vi "MB_TCP_ZERO.vi"(5 "Status Reference":T1, 6 "N":i32, 7 "Data Reference":T2, 9 "timeouts":T3={"conn_timeout"=1000, "reconn_timeout"=3000, "N attempt max"=3, "t_reset_TTL"=120000, "write_timeout"=10, "read_timeout"=500, "period"=100} {"t_reset_TTL" min=10 max=240000 step=1; "period" min=10 max=100000 step=1; "read_timeout" min=10 max=60000 step=1; "write_timeout" min=1 max=60000 step=1; "N attempt max" min=1 max=5 step=1; "reconn_timeout" min=10 max=240000 step=1; "conn_timeout" min=10 max=240000}, 10 "write enable":bool=TRUE, 11 "stop":bool) -> (0 "error out":errorcluster, 2 "errors":i32, 3 "Z3":u32)   [LabVIEW 2019, in "MB_TCP1.lvlib"]
uses:
  MB_TCP1.lvlib
  ICPCON Registers/Ctl/ICPCON Data.ctl
  ICPCON Status/Ctl/ICPCON Status.ctl
  Timer Delay/unix time 1ms.vi
  Timer Delay/Timers.lvlib
  ICPCON Registers/ICPCON Registers.lvlib
  ICPCON Status/ICPCON Status.lvlib
panel:
  out "stopped":bool
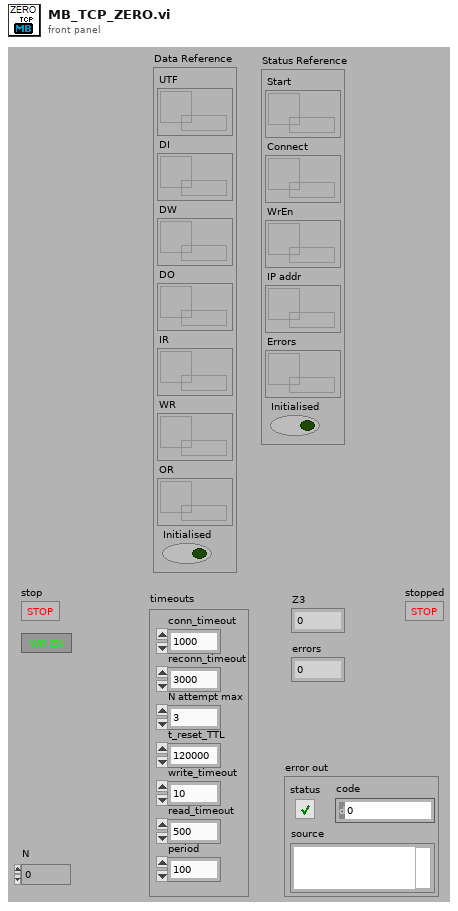
[diagram p1: front panel]
types:
  T1 = typedef "ICPCON Status.lvlib/ICPCON Status.ctl" = cluster{"Start":refnum<data-value>, "Connect":refnum<data-value>, "WrEn":refnum<data-value>, "IP addr":refnum<data-value>, "Errors":refnum<data-value>, "Initialised":bool}
  T2 = typedef "ICPCON Registers.lvlib/ICPCON Data.ctl" = cluster{"UTF":refnum<data-value>, "DI":refnum<data-value>, "DW":refnum<data-value>, "DO":refnum<data-value>, "IR":refnum<data-value>, "WR":refnum<data-value>, "OR":refnum<data-value>, "Initialised":bool}
  T3 = cluster{"conn_timeout":i32, "reconn_timeout":i32, "N attempt max":i32, "t_reset_TTL":i32, "write_timeout":i32, "read_timeout":i32, "period":i32}
  T4 = cluster{"Remote IP Address":string, "Remote Port":u16}
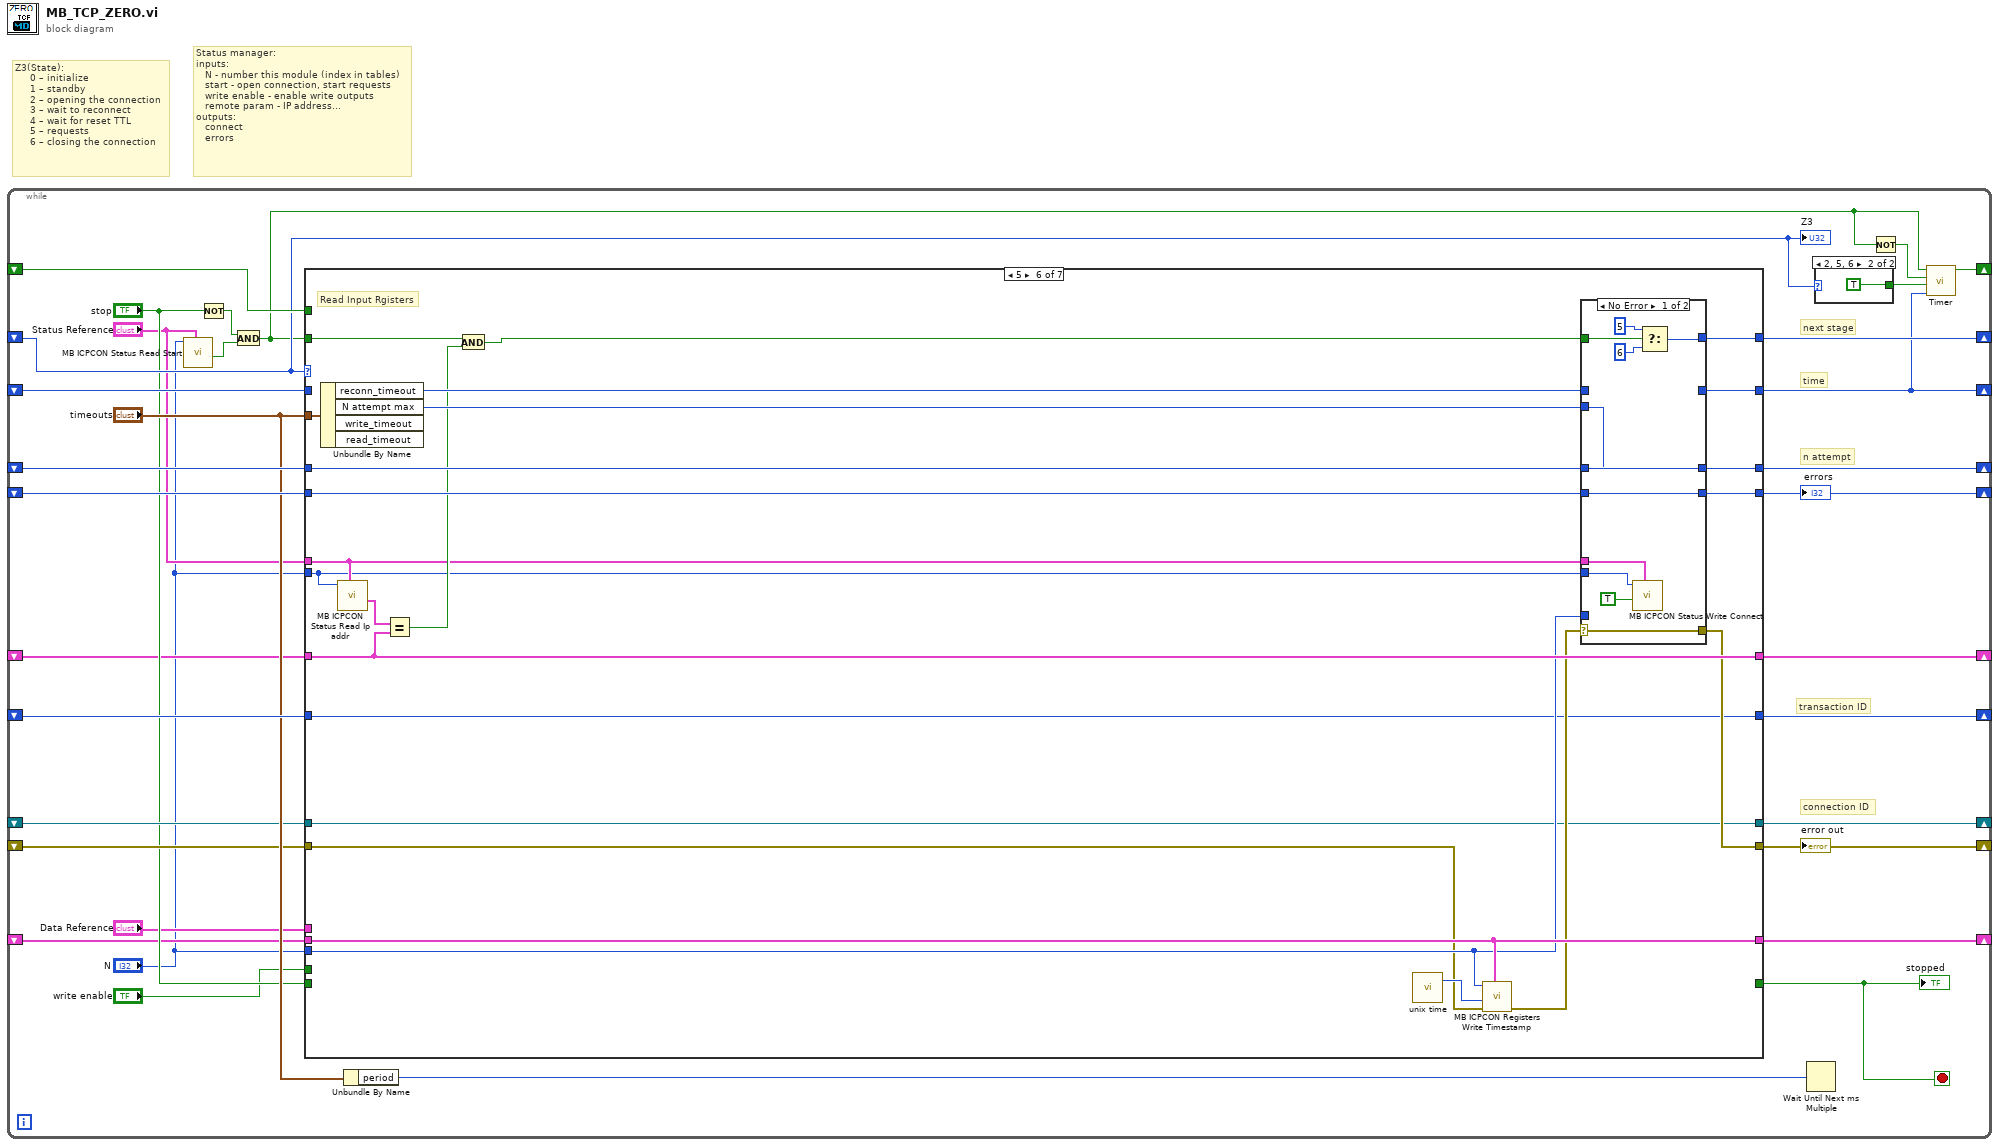
[diagram p0: block diagram]
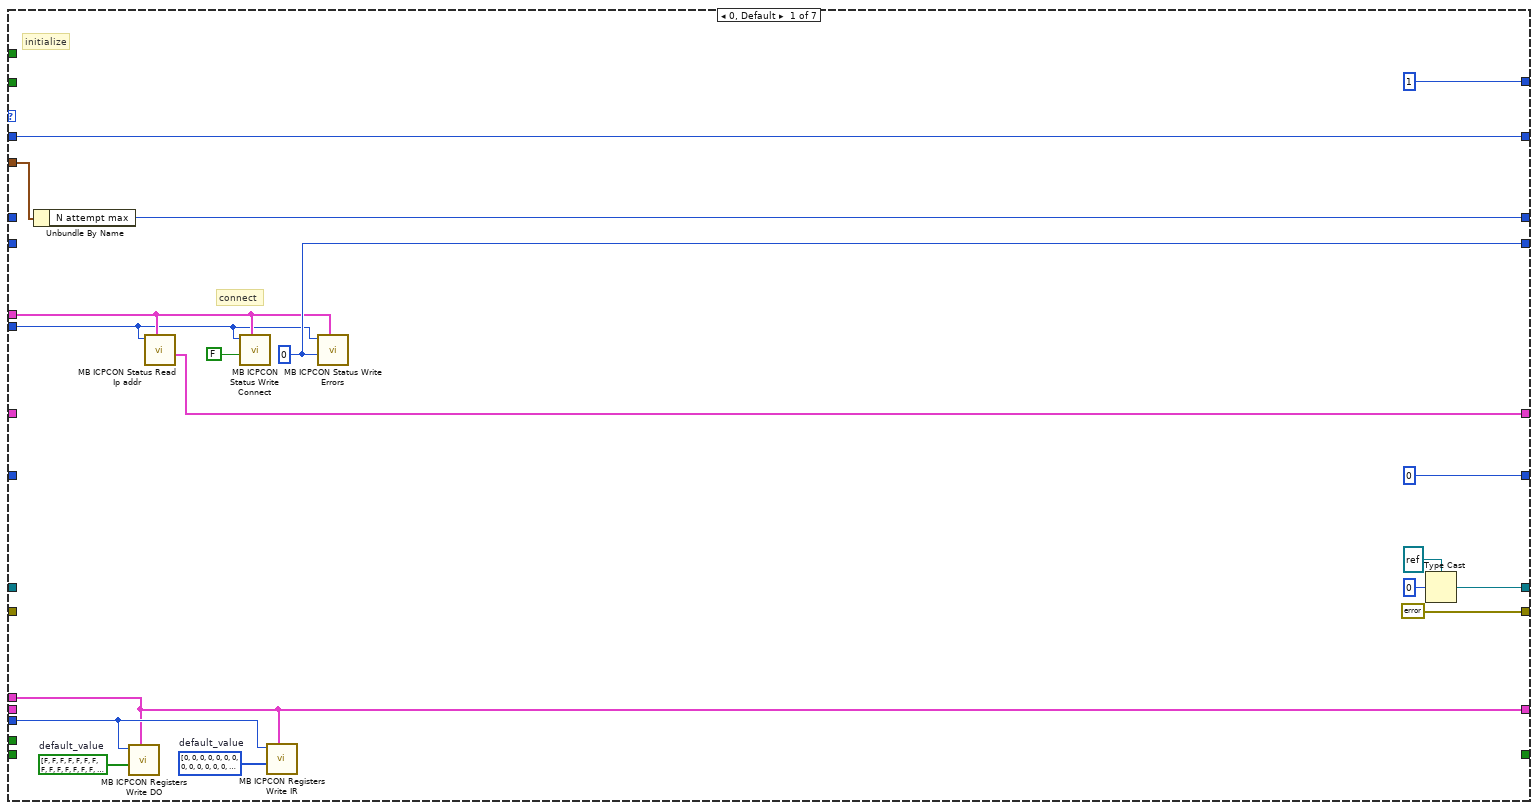
[diagram p2: hidden frame]
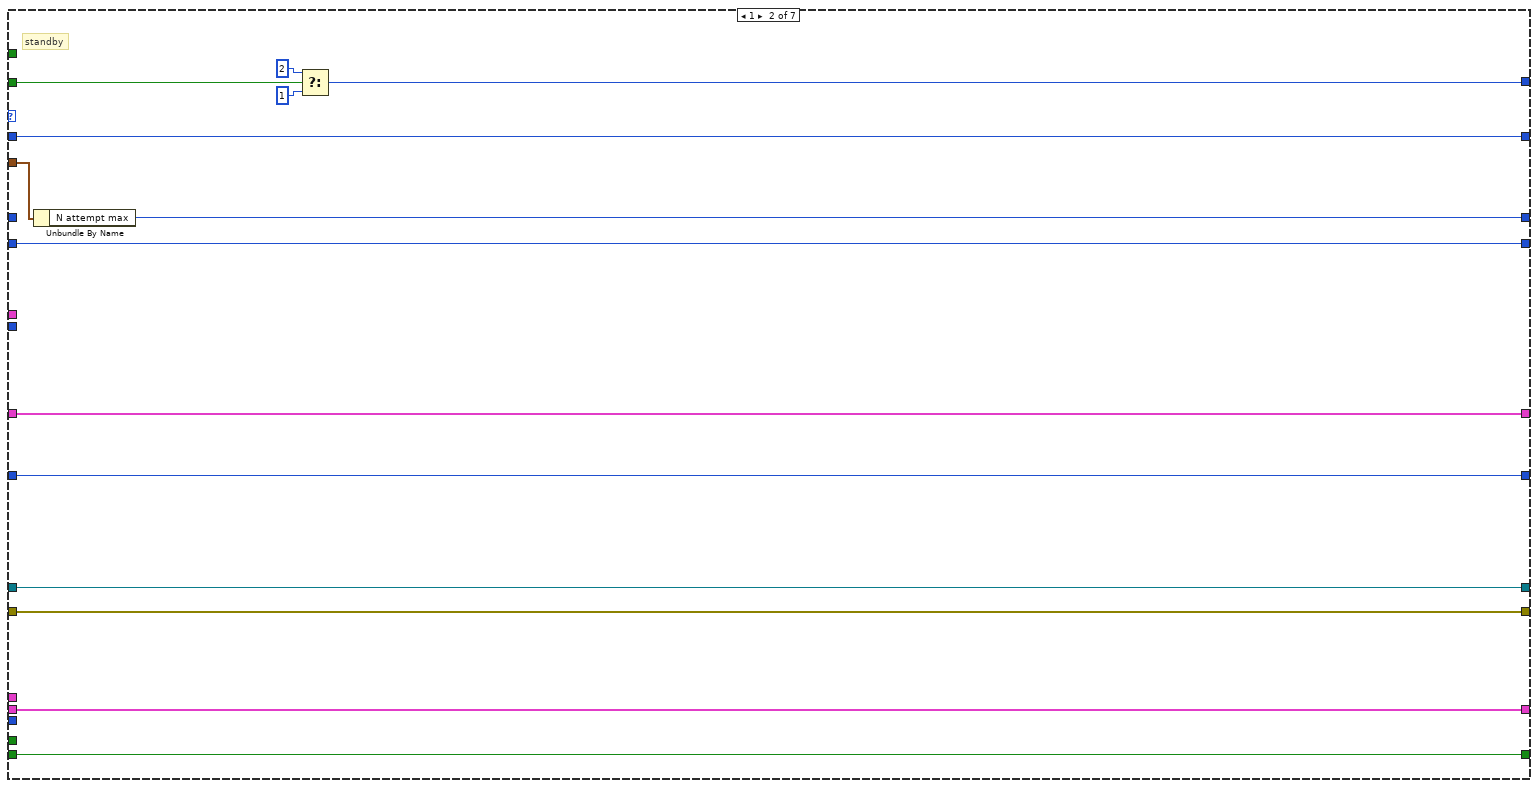
[diagram p3: hidden frame]
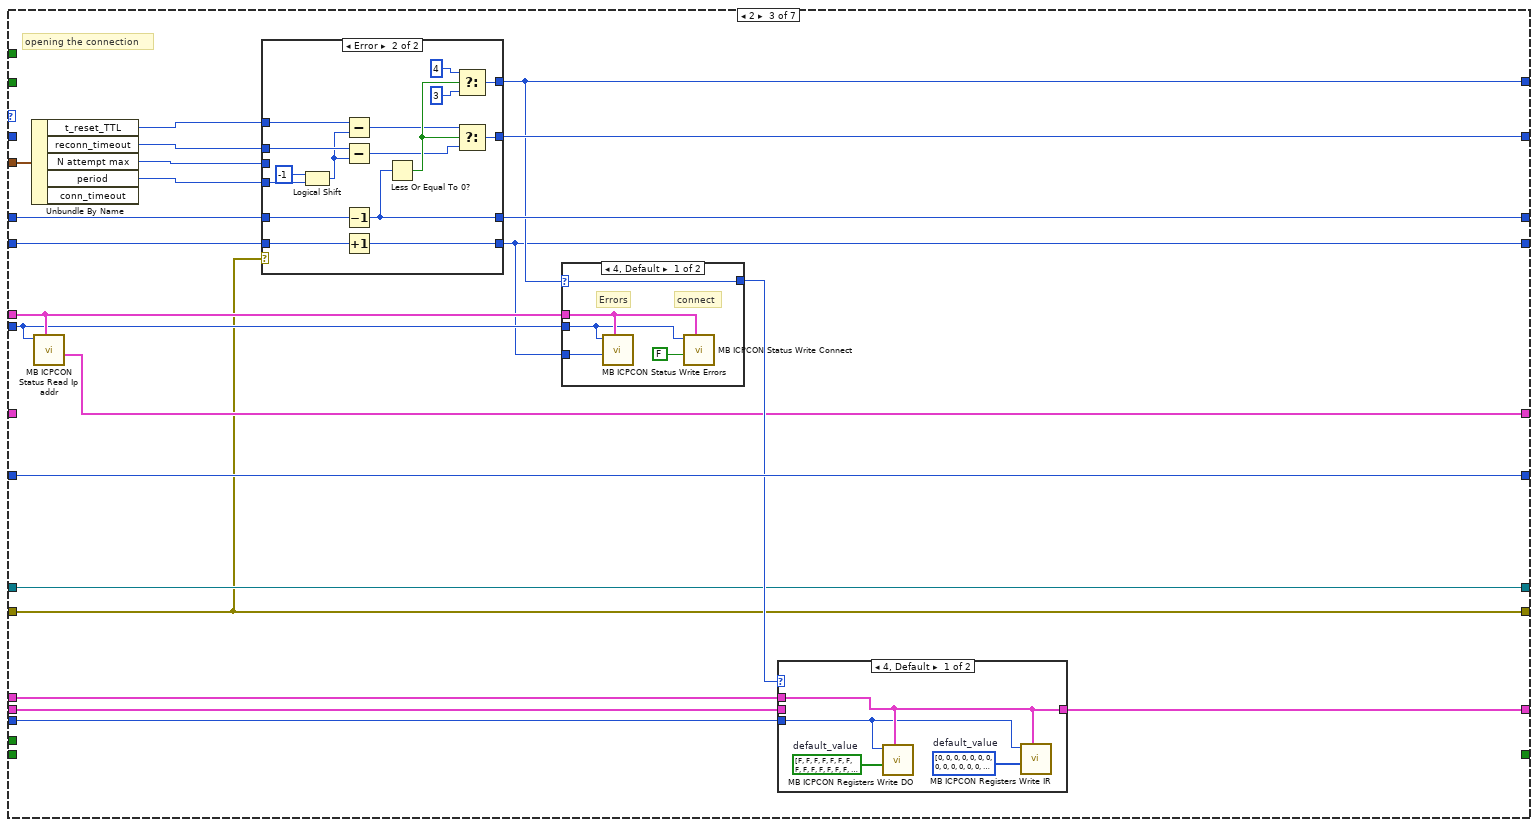
[diagram p4: hidden frame]
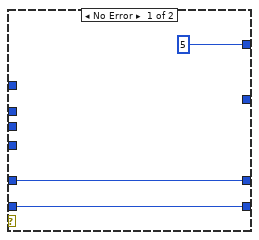
[diagram p7: hidden frame]
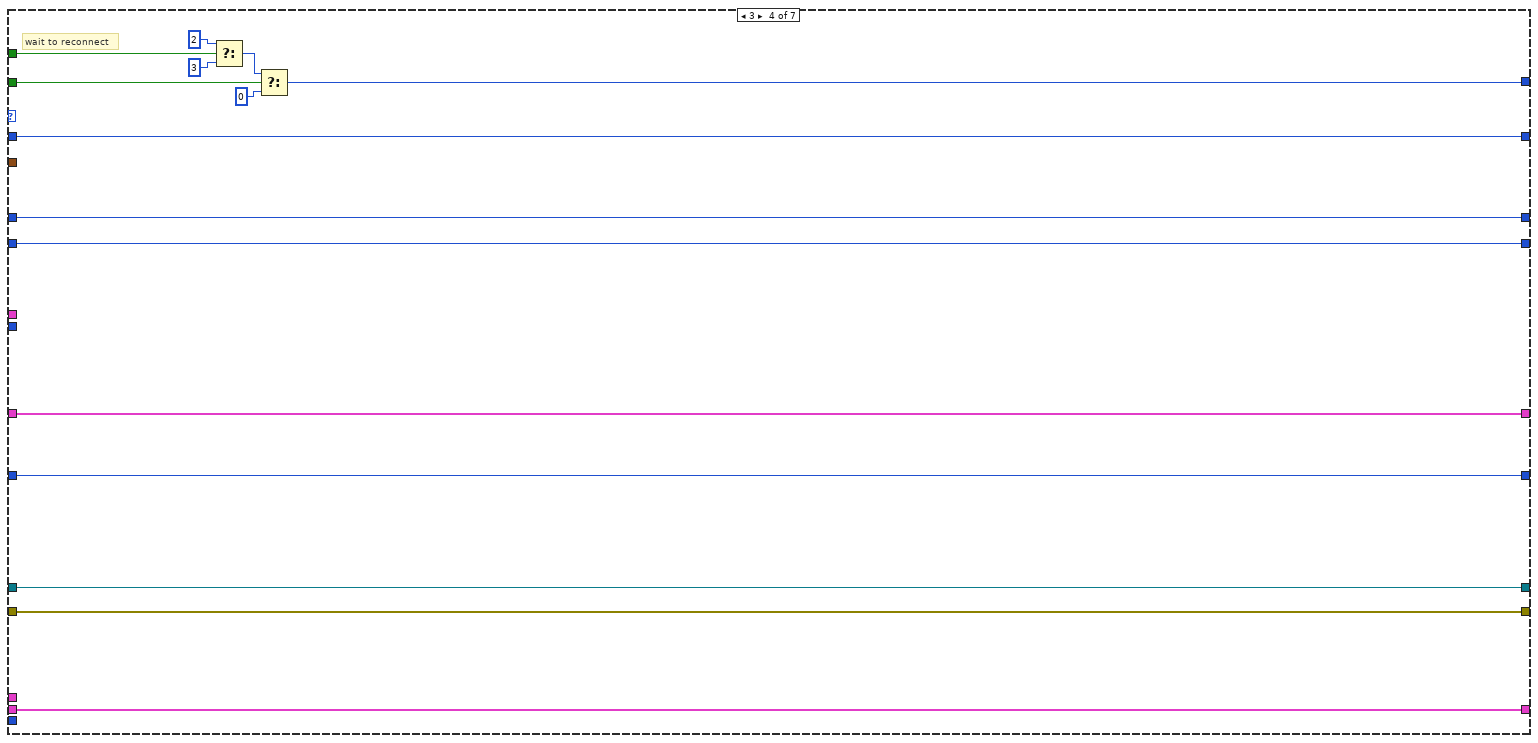
[diagram p8: hidden frame]
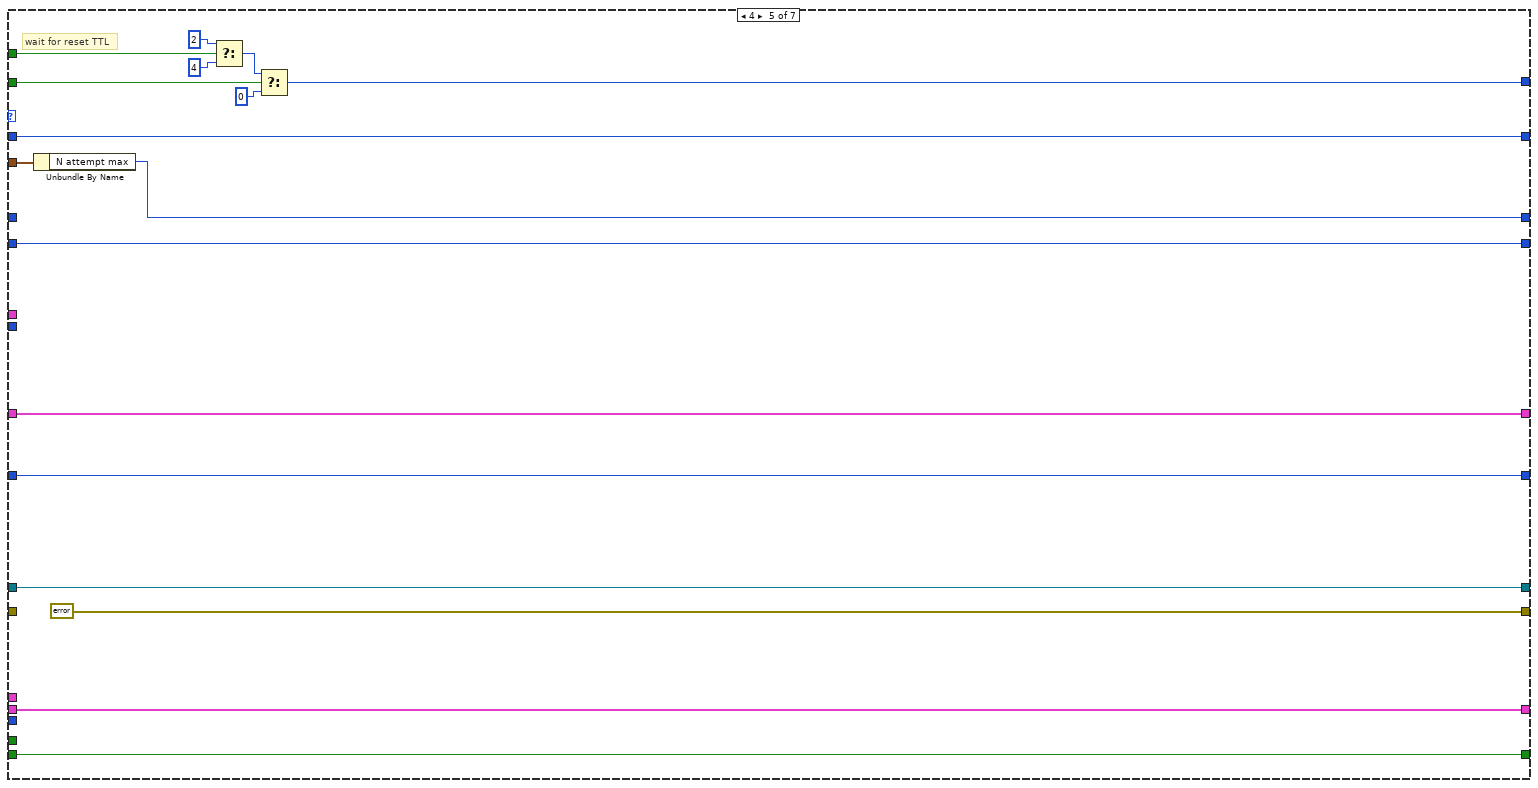
[diagram p9: hidden frame]
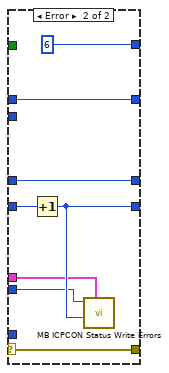
[diagram p10: hidden frame]
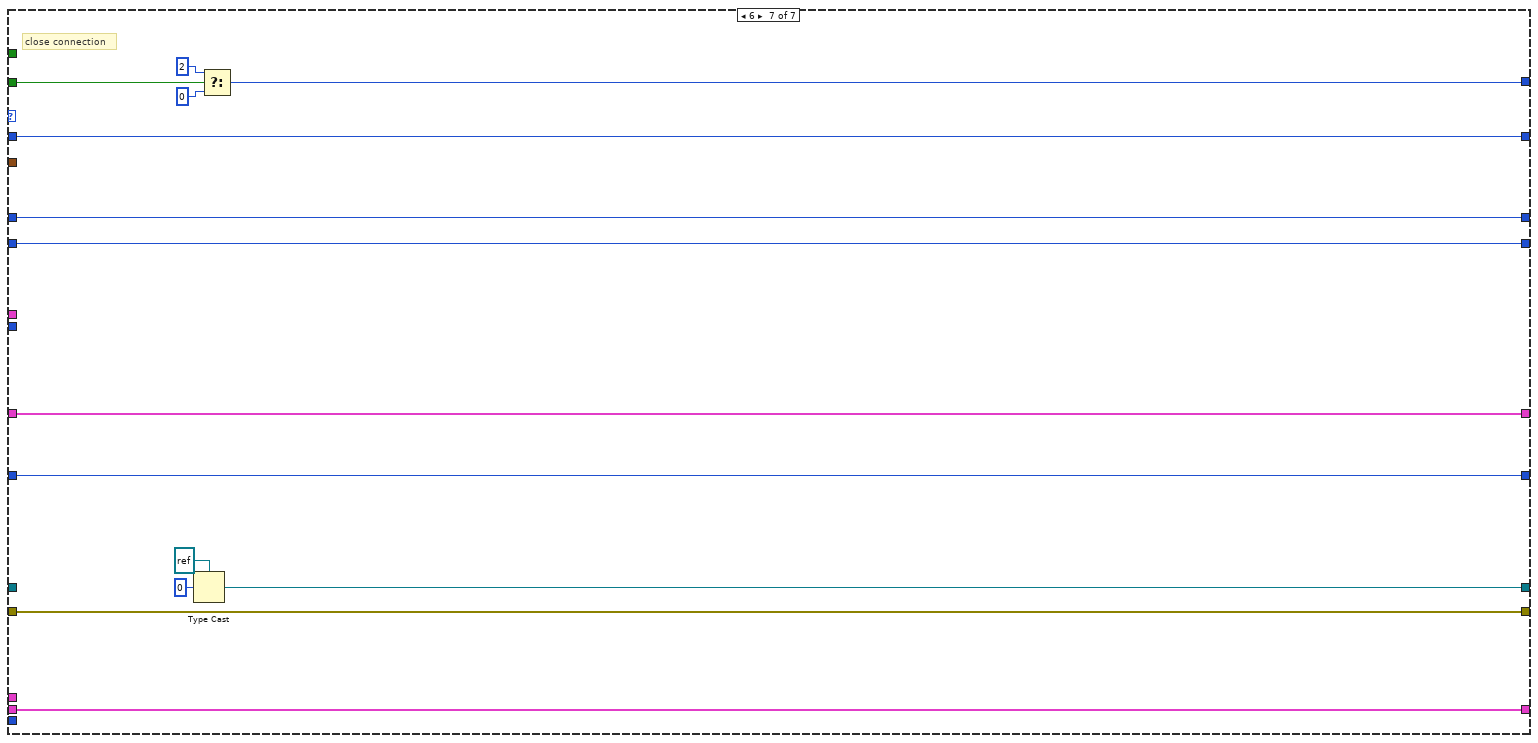
[diagram p11: hidden frame]
diagram:
  # "Status manager:\ninputs:\n   N - number this module (index in tables)\n   start - open connection, start requests\n   write enable - enable write outputs\n   remote param - IP address...\noutputs:\n   connect\n   errors"
  # "Z3(State):\n     0 – initialize \n     1 – standby\n     2 – opening the connection\n     3 – wait to reconnect\n     4 – wait for reset TTL\n     5 – requests\n     6 – closing the connection"
  n1 = while {
    shift-right: [w18] -> _
    shift-left: _ -> [w14]
    shift-right: [w17] -> _
    shift-left: _ -> [w32]
    shift-right: [w31] -> _
    shift-left: _ -> [w29]
    shift-right: [w30] -> _
    shift-left: _ -> [w28]
    shift-right: [w27] -> _
    shift-left: _ -> [w19]
    shift-right: [w26] -> _
    shift-left: _ -> [w20]
    shift-right: [w25] -> _
    shift-left: _ -> [w24]
    shift-right: [w16] -> _
    shift-left: _ -> [w15]
    shift-right: [w10] -> _
    shift-left: _ -> [w9]
    shift-right: [w7] -> _
    shift-left: _ -> [w6]
    stop <- w1 stop-if-true
    # "connection ID"
    # "transaction ID"
    # "n attempt"
    # "time"
    # "next stage"
    n2 = call "MB ICPCON Status Read Start.vi"("Status Reference"="Status Reference", "N"="N") -> ("Start"=w4:bool)  [unwired: 8 in, 1 out]
    n3 = Not(x="stop") -> (.not. x?=w12:bool)
    n4 = And(x=w12, y=w4) -> (x .and. y?=w13:bool)
    n5 = case shown="5" w14 {
      tunnel: [w49 w57 w67 w130 w135 w151 w203] -> w27
      tunnel: [errorcluster {"status"=FALSE, "code"=0, "source"=""} ("error out") w56 w66 w129 errorcluster {"status"=FALSE, "code"=0, "source"=""} ("error out") w160 w191] -> w26
      tunnel: w19 -> [_ w57 w67 w130 w135 w151 _]
      tunnel: w20 -> [_ w56 w66 w129 _ w150 w191]
      tunnel: w24 -> [_ w65 w87 w132 w149 w152 w204]
      tunnel: [u16 0 ("x") w65 w87 w132 w149 w152 w204] -> w25
      tunnel: [w44 w61 w83 w131 w145 w171 w198] -> w31
      tunnel: w29 -> [_ _ w84 w131 _ w171 w198]
      tunnel: [w36 w64 w68 w128 w148 w170 w202] -> w30
      tunnel: w28 -> [_ w64 w86 w128 w148 w169 w202]
      tunnel: [w46 w63 w80 w127 w147 w166 w201] -> w17
      tunnel: w32 -> [w46 w63 _ w127 w147 _ w201]
      tunnel: "timeouts" -> [w45 w62 w85 _ w146 w172 _]
      tunnel: w13 -> [_ w55 _ w123 w137 w164 w199]
      tunnel: [u32 1 w58 w77 w120 w140 w165 w194] -> w18
      tunnel: w15 -> [_ _ _ w121 w139 _ _]
      tunnel: "N" -> [w40 _ w74 _ _ w156 _]
      tunnel: "stop" -> [_ w54 _ _ w136 _ _]
      tunnel: [_ w54 _ _ w136 _ _] -> w1
      tunnel: [w37 w53 w71 w119 w134 w162 w193] -> w10
      tunnel: w9 -> [_ w53 _ w119 w134 w162 w193]
      tunnel: "Data Reference" -> [w39 _ w73 _ _ _ _]
      tunnel: [w39 w52 w76 w118 w133 w159 w192] -> w7
      tunnel: w6 -> [_ w52 w72 w118 w133 w159 w192]
      tunnel: "write enable" -> [_ _ _ _ _ _ _]
      tunnel: "Status Reference" -> [w35 _ w70 _ _ w154 _]
      tunnel: "N" -> [w34 _ w69 _ _ w153 _]
      frame 0, Default {
        w36 = 0 ("N attempt max")
        w41 = bool[] [FALSE, FALSE, FALSE, FALSE, FALSE, FALSE, FALSE, FALSE, FALSE, FALSE, FALSE, FALSE, FALSE, FALSE, FALSE, FALSE, FALSE, FALSE, FALSE, FALSE, FALSE, FALSE, FALSE, FALSE, FALSE, FALSE, FALSE, FALSE, FALSE, FALSE, FALSE, FALSE]  # default_value
        w42 = u16[] [0, 0, 0, 0, 0, 0, 0, 0, 0, 0, 0, 0, 0, 0, 0, 0, 0, 0, 0, 0]  # default_value
        # "connect"
        # "initialize"
        n6 = Unbundle By Name(w45) -> ("N attempt max"=w44:i32)
        n7 = call "MB ICPCON Registers Write DO.vi"("Data Reference"=w39, "Bits In"=w41, "N"=w40) -> ()  [unwired: 8 in, 1 out]
        n8 = call "MB ICPCON Status Read Ip addr.vi"("Status Reference"=w35, "N"=w34) -> ("IP address"=w37:T4)  [unwired: 8 in, 1 out]
        n9 = call "MB ICPCON Status Write Connect.vi"("Status Reference"=w35, "Connect"=FALSE ("connect"), "N"=w34) -> ()  [unwired: 8 in, 1 out]
        n10 = call "MB ICPCON Registers Write IR.vi"("Data Reference"=w39, "Words In"=w42, "N"=w40) -> ()  [unwired: 8 in, 1 out]
        n11 = call "MB ICPCON Status Write Errors.vi"("Status Reference"=w35, "Errors"=w36, "N"=w34) -> ()  [unwired: 8 in, 1 out]
        n12 = Type Cast(type=refnum<k5> refnum ("connection ID"), x=u32 0) -> (*(type *) &x=w49:refnum<k5>)
      }
      frame 1 {
        # "standby"
        n13 = Unbundle By Name(w62) -> ("N attempt max"=w61:i32)
        n14 = Select(t=u32 2, s=w55, f=u32 1) -> (s? t:f=w58:u32)
      }
      frame 2 {
        # "opening the connection"
        n15 = Unbundle By Name(w85) -> ("t_reset_TTL"=w79:i32, "reconn_timeout"=w81:i32, "N attempt max"=w82:i32, "period"=w78:i32)  [unwired: 1 out]
        n16 = call "MB ICPCON Status Read Ip addr.vi"("Status Reference"=w70, "N"=w69) -> ("IP address"=w71:T4)  [unwired: 8 in, 1 out]
        n17 = case shown="Error" w66 {
          tunnel: w86 -> [w101 w117]
          tunnel: [w101 w116] -> w68
          tunnel: w84 -> [w100 w115]
          tunnel: [w100 w114] -> w83
          tunnel: w82 -> [_ _]
          tunnel: [u32 5 w111] -> w77
          tunnel: w81 -> [_ w110]
          tunnel: [_ w109] -> w80
          tunnel: w79 -> [_ w106]
          tunnel: w78 -> [_ w104]
          frame No Error {
          }
          frame Error {
            n18 = Logical Shift(y=i16 -1, x=w104) -> (x << y=w102:i32)
            n19 = Subtract(x=w106, y=w102) -> (x-y=w105:i32)
            n20 = Subtract(x=w110, y=w102) -> (x-y=w107:i32)
            n21 = Decrement(x=w115) -> (x-1=w114:i32)
            n22 = Increment(x=w117) -> (x+1=w116:i32)
            n23 = Less Or Equal To 0?(x=w114) -> (x <= 0?=w108:bool)
            n24 = Select(t=u32 4, s=w108, f=u32 3) -> (s? t:f=w111:u32)
            n25 = Select(t=w105, s=w108, f=w107) -> (s? t:f=w109:i32)
          }
        }
        n26 = case shown="4, Default" w77 {
          selector: w77 -> [w97 w98]
          tunnel: [w97 w98] -> w75
          tunnel: w70 -> [w95 _]
          tunnel: w69 -> [w94 _]
          tunnel: w68 -> [w93 _]
          frame 4, Default {
            # "Errors"
            # "connect"
            n27 = call "MB ICPCON Status Write Errors.vi"("Status Reference"=w95, "Errors"=w93, "N"=w94) -> ()  [unwired: 8 in, 1 out]
            n28 = call "MB ICPCON Status Write Connect.vi"("Status Reference"=w95, "Connect"=FALSE ("f"), "N"=w94) -> ()  [unwired: 8 in, 1 out]
          }
          frame 3, 5 {
          }
        }
        n29 = case shown="4, Default" w75 {
          tunnel: w74 -> [w88 _]
          tunnel: w72 -> [_ w92]
          tunnel: [w89 w92] -> w76
          tunnel: w73 -> [w89 _]
          frame 4, Default {
            w90 = bool[] [FALSE, FALSE, FALSE, FALSE, FALSE, FALSE, FALSE, FALSE, FALSE, FALSE, FALSE, FALSE, FALSE, FALSE, FALSE, FALSE, FALSE, FALSE, FALSE, FALSE, FALSE, FALSE, FALSE, FALSE, FALSE, FALSE, FALSE, FALSE, FALSE, FALSE, FALSE, FALSE]  # default_value
            w91 = u16[] [0, 0, 0, 0, 0, 0, 0, 0, 0, 0, 0, 0, 0, 0, 0, 0, 0, 0, 0, 0]  # default_value
            n30 = call "MB ICPCON Registers Write DO.vi"("Data Reference"=w89, "Bits In"=w90, "N"=w88) -> ()  [unwired: 8 in, 1 out]
            n31 = call "MB ICPCON Registers Write IR.vi"("Data Reference"=w89, "Words In"=w91, "N"=w88) -> ()  [unwired: 8 in, 1 out]
          }
          frame 3, 5 {
          }
        }
      }
      frame 3 {
        # "wait to reconnect"
        n32 = Select(t=u32 2, s=w121, f=u32 3) -> (s? t:f=w122:u32)
        n33 = Select(t=w122, s=w123, f=u32 0) -> (s? t:f=w120:u32)
      }
      frame 4 {
        # "wait for reset TTL"
        n34 = Unbundle By Name(w146) -> ("N attempt max"=w145:i32)
        n35 = Select(t=u32 2, s=w139, f=u32 4) -> (s? t:f=w141:u32)
        n36 = Select(t=w141, s=w137, f=u32 0) -> (s? t:f=w140:u32)
      }
      frame 5 {
        # "Read Input Rgisters"
        n37 = Unbundle By Name(w172) -> ("reconn_timeout"=w167:i32, "N attempt max"=w168:i32)  [unwired: 2 out]
        n38 = call "MB ICPCON Status Read Ip addr.vi"("Status Reference"=w154, "N"=w153) -> ("IP address"=w155:T4)  [unwired: 8 in, 1 out]
        n39 = Equal?(x=w155, y=w162) -> (x = y?=w161:bool)
        n40 = And(x=w164, y=w161) -> (x .and. y?=w163:bool)
        n41 = call-poly "unix time.vi"() -> ("unix time (ms)"=w157:u64)  [unwired: 2 in, 1 out]
        n42 = call "MB ICPCON Registers Write Timestamp.vi"("Data Reference"=w159, "error in (no error)"=w150, "UTF"=w157, "N"=w156) -> ("error out"=w158:errorcluster)  [unwired: 7 in]
        n43 = case shown="No Error" w158 {
          selector: w158 -> [w176 w186]
          tunnel: w169 -> [w177 w190]
          tunnel: [w177 w185] -> w170
          tunnel: [w179 u32 6] -> w165
          tunnel: w171 -> [_ w188]
          tunnel: w168 -> [w182 _]
          tunnel: [w182 w188] -> _
          tunnel: w167 -> [_ w187]
          tunnel: [_ w187] -> w166
          tunnel: w163 -> [w178 _]
          tunnel: w156 -> [_ _]
          tunnel: [w176 w186] -> w160
          tunnel: w154 -> [w174 w184]
          tunnel: w153 -> [w173 w183]
          frame No Error {
            n44 = call "MB ICPCON Status Write Connect.vi"("Status Reference"=w174, "Connect"=TRUE ("f"), "N"=w173) -> ()  [unwired: 8 in, 1 out]
            n45 = Select(t=u32 5, s=w178, f=u32 6) -> (s? t:f=w179:u32)
          }
          frame Error {
            n46 = Increment(x=w190) -> (x+1=w185:i32)
            n47 = call "MB ICPCON Status Write Errors.vi"("Status Reference"=w184, "Errors"=w185, "N"=w183) -> ()  [unwired: 8 in, 1 out]
          }
        }
      }
      frame 6 {
        # "close connection"
        n48 = Type Cast(type=refnum<k5> refnum ("connection ID"), x=u32 0) -> (*(type *) &x=w203:refnum<k5>)
        n49 = Select(t=u32 2, s=w199, f=u32 0) -> (s? t:f=w194:u32)
      }
    }
    "error out" <- w26
    "errors" <- w30
    "stopped" <- w1
    n50 = Unbundle By Name("timeouts") -> ("period"=w22:i32)
    n51 = Wait Until Next ms Multiple(millisecond multiple=w22) -> ()  [unwired: 1 out]
    n52 = case shown="2, 5, 6" w14 {
      tunnel: [_ TRUE] -> w21
      frame 0, Default {
      }
      frame 2, 5, 6 {
      }
    }
    n53 = Not(x=w13) -> (.not. x?=w33:bool)
    n54 = call "Timer.vi"("ms"=w17, "Load (F)"=w21, "Reset (F)"=w33, "Start (T)"=w13) -> ("End"=w16:bool)  [unwired: 5 in, 1 out]
    "Z3" <- w14
  }
